vi "downloading_data.vi"(8 "maxDistance":string) -> (0 "Historical indexes":map{string, variant}[](array[numeric]), 1 "Historical standards":map{string, i32}[](array[numeric]), 2 "Current standards [%]":map{string, i32}(c390), 3 "Current indexes":map{string, variant}(c390), 4 "Historical conditions":map{string, i32}[](array[numeric]), 5 "Current conditions":map{string, i32}(c390), 6 "Historical timestamps":map{string, string}[](array[numeric]), 7 "Current timestamps":map{string, string}(c390))   [LabVIEW 2019]
uses:
  <vilib>/Utility/NIReport.llb/Report Type.ctl
  <vilib>/LVH/i3 JSON/JSON Parsing/Get Object Parameter Files/Get Object Parameter - Object.vi
  <vilib>/LVH/i3 JSON/JSON Parsing/Get Object Parameter Files/Get Object Parameter - Array.vi
  <vilib>/LVH/i3 JSON/JSON Parsing/Get Array Value at Index Files/Get Array Value at Index - Object.vi
  <vilib>/Utility/NIReport.llb/NI_report.lvclass
  <vilib>/httpClient/LabVIEWHTTPClient.lvlib
  <vilib>/LVH/i3 JSON/i3-json.lvlib
  <vilib>/Utility/NIReport.llb/NI_ReportGenerationCore.lvlib
  <vilib>/Utility/NIReport.llb/Word/NI_Word.lvclass
panel:
  out "wartości":i32[](array[numeric])
  in  "Window State 2":enum16{"maximized", "minimized", "normal"}(ring)
  in  "Month 2":string[](array[string])=["Jan", "Feb", "Mar", "Apr", "May"]
  in  "Graph Type 2":i32(ring)=51 items=["xlColumnClustered"=51, "xlColumnStacked"=52, "xlColumnStacked100"=53, "xl3DColumnClustered"=54, "xl3DColumnStacked"=55, "xl3DColumnStacked100"=56, "xlBarClustered"=57, "xlBarStacked"=58, "xlBarStacked100"=59, "xl3DBarClustered"=60, "xl3DBarStacked"=61, "xl3DBarStacked100"=62, "xlLineStacked"=63, "xlLineStacked100"=64, "xlLineMarkers"=65, "xlLineMarkersStacked"=66, "xlLineMarkersStacked100"=67, "xlPieOfPie"=68, "xlPieExploded"=69, "xl3DPieExploded"=70, "xlBarOfPie"=71, "xlXYScatterSmooth"=72, "xlXYScatterSmoothNoMarkers"=73, "xlXYScatterLines"=74, "xlXYScatterLinesNoMarkers"=75, "xlAreaStacked"=76, "xlAreaStacked100"=77, "xl3DAreaStacked"=78, "xl3DAreaStacked100"=79, "xlDoughnutExploded"=80, "xlRadarMarkers"=81, "xlRadarFilled"=82, "xlSurface"=83, "xlSurfaceWireframe"=84, "xlSurfaceTopView"=85, "xlSurfaceTopViewWireframe"=86, "xlBubble"=15, "xlBubble3DEffect"=87, "xlStockHLC"=88, "xlStockOHLC"=89, "xlStockVHLC"=90, "xlStockVOHLC"=91, "xlCylinderColClustered"=92, "xlCylinderColStacked"=93, "xlCylinderColStacked100"=94, "xlCylinderBarClustered"=95, "xlCylinderBarStacked"=96, "xlCylinderBarStacked100"=97, "xlCylinderCol"=98, "xlConeColClustered"=99, "xlConeColStacked"=100, "xlConeColStacked100"=101, "xlConeBarClustered"=102, "xlConeBarStacked"=103, "xlConeBarStacked100"=104, "xlConeCol"=105, "xlPyramidColClustered"=106, "xlPyramidColStacked"=107, "xlPyramidColStacked100"=108, "xlPyramidBarClustered"=109, "xlPyramidBarStacked"=110, "xlPyramidBarStacked100"=111, "xlPyramidCol"=112, "xl3DColumn"=-4100, "xlLine"=4, "xl3DLine"=-4101, "xl3DPie"=-4102, "xlPie"=5, "xlXYScatter"=-4169, "xl3DArea"=-4098, "xlArea"=1, "xlDoughnut"=-4120, "xlRadar"=-4151]
  in  "Has Legend? 2":bool
  in  "Relative Humidity 2":dbl[][](array[numeric])=[[0.54, 0.65, 0.56, 0.5, 0.45]]
  in  "Window State":enum16{"maximized", "minimized", "normal"}(ring)
  in  "Month":string[](array[string])=["Jan", "Feb", "Mar", "Apr", "May"]
  in  "Graph Type":i32(ring)=51 items=["xlColumnClustered"=51, "xlColumnStacked"=52, "xlColumnStacked100"=53, "xl3DColumnClustered"=54, "xl3DColumnStacked"=55, "xl3DColumnStacked100"=56, "xlBarClustered"=57, "xlBarStacked"=58, "xlBarStacked100"=59, "xl3DBarClustered"=60, "xl3DBarStacked"=61, "xl3DBarStacked100"=62, "xlLineStacked"=63, "xlLineStacked100"=64, "xlLineMarkers"=65, "xlLineMarkersStacked"=66, "xlLineMarkersStacked100"=67, "xlPieOfPie"=68, "xlPieExploded"=69, "xl3DPieExploded"=70, "xlBarOfPie"=71, "xlXYScatterSmooth"=72, "xlXYScatterSmoothNoMarkers"=73, "xlXYScatterLines"=74, "xlXYScatterLinesNoMarkers"=75, "xlAreaStacked"=76, "xlAreaStacked100"=77, "xl3DAreaStacked"=78, "xl3DAreaStacked100"=79, "xlDoughnutExploded"=80, "xlRadarMarkers"=81, "xlRadarFilled"=82, "xlSurface"=83, "xlSurfaceWireframe"=84, "xlSurfaceTopView"=85, "xlSurfaceTopViewWireframe"=86, "xlBubble"=15, "xlBubble3DEffect"=87, "xlStockHLC"=88, "xlStockOHLC"=89, "xlStockVHLC"=90, "xlStockVOHLC"=91, "xlCylinderColClustered"=92, "xlCylinderColStacked"=93, "xlCylinderColStacked100"=94, "xlCylinderBarClustered"=95, "xlCylinderBarStacked"=96, "xlCylinderBarStacked100"=97, "xlCylinderCol"=98, "xlConeColClustered"=99, "xlConeColStacked"=100, "xlConeColStacked100"=101, "xlConeBarClustered"=102, "xlConeBarStacked"=103, "xlConeBarStacked100"=104, "xlConeCol"=105, "xlPyramidColClustered"=106, "xlPyramidColStacked"=107, "xlPyramidColStacked100"=108, "xlPyramidBarClustered"=109, "xlPyramidBarStacked"=110, "xlPyramidBarStacked100"=111, "xlPyramidCol"=112, "xl3DColumn"=-4100, "xlLine"=4, "xl3DLine"=-4101, "xl3DPie"=-4102, "xlPie"=5, "xlXYScatter"=-4169, "xl3DArea"=-4098, "xlArea"=1, "xlDoughnut"=-4120, "xlRadar"=-4151]
  out "nagłówki":string[](array[string])
  out "longitude":string
  out "latitude":string
  out "Latitude":dbl
  out "Longitude":dbl
  in  "Tab":enum32{"Current", "Historical"}(tab)
  out "body":string
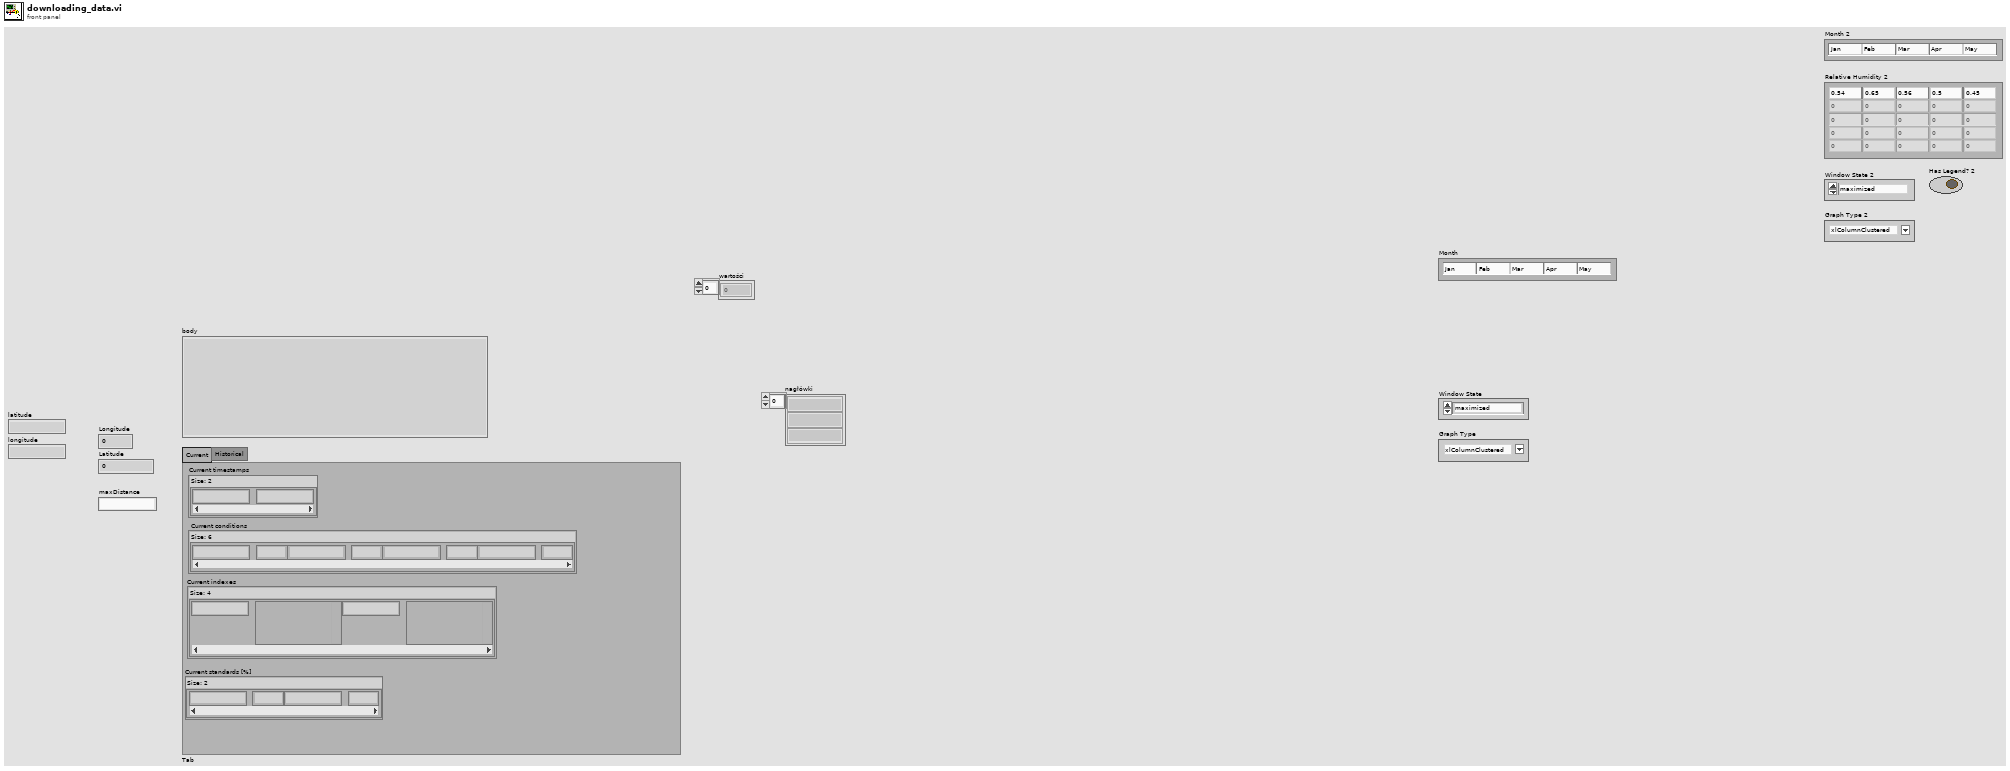
[diagram p1: front panel]
types:
  T1 = cluster{"font style":string, "bold":bool, "italic":bool, "underline":bool, "size":sgl, "color":u32}
  T2 = typedef "NI_ReportGenerationCore.lvlib/Report Type.ctl" = enum16{"HTML", "Word", "Excel"}
  T3 = cluster{"current":cluster{"fromDateTime":string, "tillDateTime":string, "values":cluster{"type and defaults":cluster{"name":string, "value":dbl}, "type and defaults 2":cluster{"name":string, "value":dbl}, "type and defaults 3":cluster{"name":string, "value":dbl}, "type and defaults 4":cluster{"name":string, "value":dbl}, "type and defaults 5":cluster{"name":string, "value":dbl}, "type and defaults 6":cluster{"name":string, "value":dbl}}, "indexes":cluster{"type and defaults":cluster{"name":string, "value":dbl, "level":string, "description":string, "advice":string, "color":string}}, "standards":cluster{"type and defaults":cluster{"name":string, "limit":dbl, "pollutant":string, "percent":dbl}, "type and defaults 2":cluster{"name":string, "limit":dbl, "pollutant":string, "percent":dbl}}}}
  T4 = typedef "LabVIEWHTTPClient.lvlib/ClientHandle.ctl" = refnum<k1>
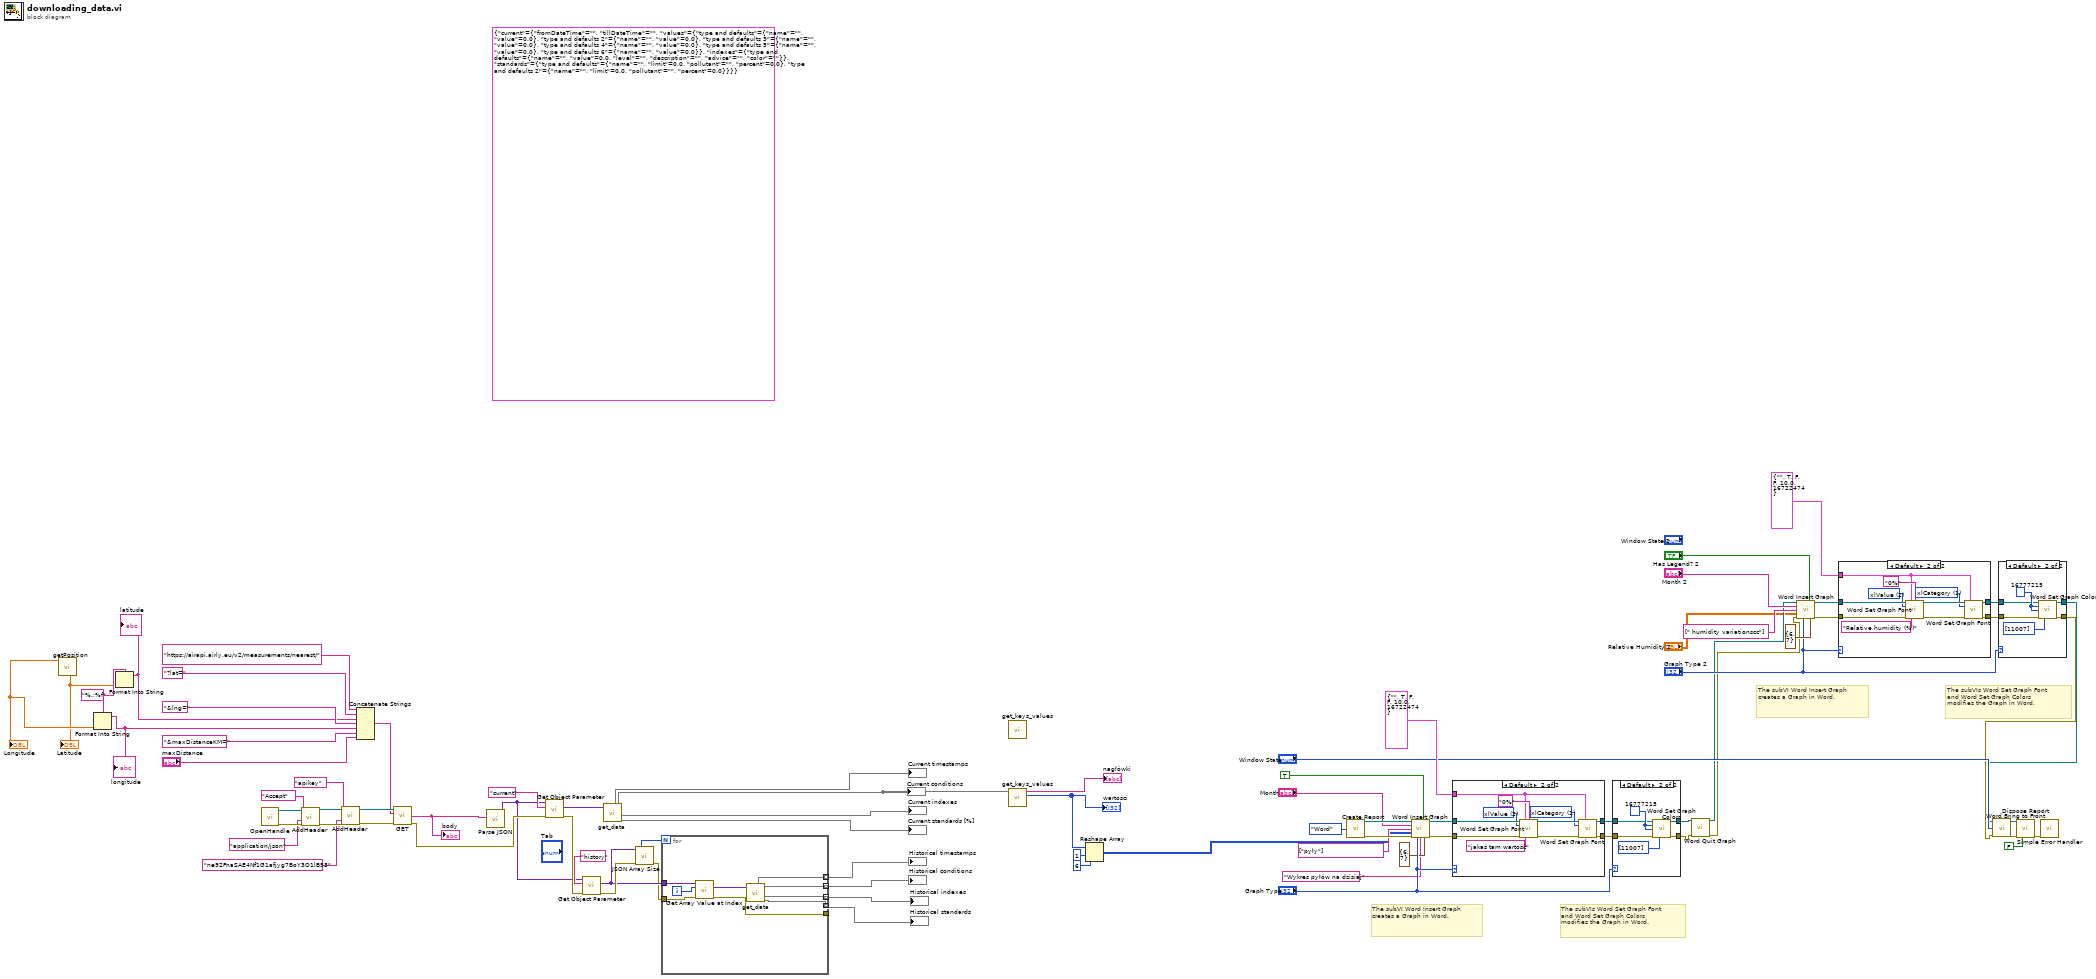
[diagram p0: block diagram]
diagram:
  w45 = "%.;%f" ("format string")
  (unwired) T3 {"current"={"fromDateTime"="", "tillDateTime"="", "values"={"type and defaults"={"name"="", "value"=0.0}, "type and defaults 2"={"name"="", "value"=0.0}, "type and defaults 3"={"name"="", "value"=0.0}, "type and defaults 4"={"name"="", "value"=0.0}, "type and defaults 5"={"name"="", "value"=0.0}, "type and defaults 6"={"name"="", "value"=0.0}}, "indexes"={"type and defaults"={"name"="", "value"=0.0, "level"="", "description"="", "advice"="", "color"=""}}, "standards"={"type and defaults"={"name"="", "limit"=0.0, "pollutant"="", "percent"=0.0}, "type and defaults 2"={"name"="", "limit"=0.0, "pollutant"="", "percent"=0.0}}}} ("type and defaults")
  # "The subVIs Word Set Graph Font \nand Word Set Graph Colors \nmodifies the Graph in Word."
  # "The subVI Word Insert Graph \ncreates a Graph in Word."
  # "The subVIs Word Set Graph Font \nand Word Set Graph Colors \nmodifies the Graph in Word."
  # "The subVI Word Insert Graph \ncreates a Graph in Word."
  n1 = call "getPosition.vi"() -> ("Latitude"=w44:dbl, "Longitude"=w47:dbl)  [unwired: 10 in]
  "Longitude" <- w47
  "Latitude" <- w44
  n2 = Format Into String(format string=w45, w47) -> (resulting string=w48:string)  [unwired: 2 in, 1 out]
  "longitude" <- w48
  n3 = Format Into String(format string=w45, w44) -> (resulting string=w46:string)  [unwired: 2 in, 1 out]
  "latitude" <- w46
  n4 = call <vilib>:"OpenHandle.vi"() -> ("client handle out"=w81:T4, "error out"=w78:errorcluster)  [unwired: 14 in]
  n5 = call <vilib>:"AddHeader.vi"("client handle"=w81, "header"="Accept", "value"="application/json", "error in (no error)"=w78) -> ("client handle out"=w80:T4, "error out"=w77:errorcluster)  [unwired: 10 in]
  n6 = call <vilib>:"AddHeader.vi"("client handle"=w80, "header"="apikey", "value"="ne92FnaSAE4Nf1G1afjyg7BoY3O1lB53", "error in (no error)"=w77) -> ("client handle out"=w79:T4, "error out"=w76:errorcluster)  [unwired: 10 in]
  n7 = Concatenate Strings("https://airapi.airly.eu/v2/measurements/nearest/" ("url"), "?lat=" ("string"), w46, "&lng=" ("string"), w48, "&maxDistanceKM=" ("string"), "maxDistance") -> (w71:string)
  n8 = call <vilib>:"GET.vi"("client handle"=w79, "url"=w71, "error in (no error)"=w76) -> ("body"=w65:string, "error out"=w63:errorcluster)  [unwired: 9 in, 2 out]
  "body" <- w65
  n9 = call <vilib>:"Parse JSON.vi"("JSON String"=w65) -> ("JSON Tree"=w54:variant)  [unwired: 7 in, 3 out]
  n10 = call-poly <vilib>:"Get Object Parameter.vi"("error in (no error)"=w63, "Parameter Name"="current", "JSON Tree In (JSON Object)"=w54) -> ("error out"=w60:errorcluster, "JSON Object"=w61:variant)  [unwired: 5 in, 2 out]
  n11 = call-poly <vilib>:"Get Object Parameter.vi"("error in (no error)"=w60, "Parameter Name"="history", "JSON Tree In (JSON Object)"=w54) -> ("error out"=w58:errorcluster, "JSON Array"=w56:variant)  [unwired: 5 in, 2 out]
  n12 = call "get_data.vi"("JSON"=w61) -> ("Standards [%]"=→"Current standards [%]":map{string, i32}, "Indexes"=→"Current indexes":map{string, variant}, "Conditions"=w7:map{string, i32}, "Timestamps"=→"Current timestamps":map{string, string})  [unwired: 7 in]
  "Current conditions" <- w7
  n13 = call <vilib>:"JSON Array Size.vi"("error in (no error)"=w58, "JSON Tree In (JSON Array)"=w56) -> ("error out"=w55:errorcluster, "Array Size"=w59:i32)  [unwired: 7 in, 1 out]
  n14 = for {
    N: w59 -> [_]
    tunnel: w56 -> [w90]
    tunnel: [w87] -> w53 mode=indexing
    tunnel: [w86] -> w52 mode=indexing
    tunnel: [w85] -> w51 mode=indexing
    tunnel: [w84] -> w57 mode=indexing
    tunnel: w55 -> [w83]
    tunnel: [w82] -> _
    i -> [w89]
    n15 = call-poly <vilib>:"Get Array Value at Index.vi"("error in (no error)"=w83, "Index"=w89, "JSON Tree In (JSON Array)"=w90) -> ("error out"=w82:errorcluster, "JSON Object"=w88:variant)  [unwired: 5 in, 2 out]
    n16 = call "get_data.vi"("JSON"=w88) -> ("Standards [%]"=w85:map{string, i32}, "Indexes"=w86:map{string, variant}, "Conditions"=w87:map{string, i32}, "Timestamps"=w84:map{string, string})  [unwired: 7 in]
  }
  "Historical timestamps" <- w57
  "Historical conditions" <- w53
  "Historical indexes" <- w52
  "Historical standards" <- w51
  n17 = call "get_keys_values.vi"("Conditions"=w7) -> ("wartosci"=w5:i32[], "naglowki"=→"nagłówki":string[])  [unwired: 9 in]
  "wartości" <- w5
  n18 = call "get_keys_values.vi"() -> ()  [unwired: 10 in, 2 out]
  n19 = Reshape Array(w5, 1 ("dimension size"), 6 ("dimension size")) -> (w2:i32[][])
  n20 = call <vilib>:"Create Report.vi"("report type"=Report_Type."Word" ("Report Type")) -> ("report out"=w32:refnum<class "NI_report.lvclass">, "error out"=w33:errorcluster)  [unwired: 13 in]
  n21 = call <vilib>:"Word Insert Graph.vi"("report in"=w32, "has legend? (F)"=TRUE ("Has Legend?"), "column headers"="Month", "row headers"=string[] ["pyły"], "data"=w2, "error in (no error)"=w33, "graph type (col clustered)"="Graph Type", "graph title (\"\")"="Wykres pyłów na dzisiaj" ("graph title (\"\")"), "graph size (5, 5)"=cluster{"height":i32, "width":i32} {"height"=6, "width"=7}) -> ("report out"=w37:refnum<class "NI_report.lvclass">, "error out"=w36:errorcluster)  [unwired: 3 in, 2 out]
  n22 = case shown="Default" "Graph Type" {
    tunnel: w37 -> [w92 w103]
    tunnel: w36 -> [w91 w102]
    tunnel: [w92 w100] -> w34
    tunnel: [w91 w99] -> w35
    tunnel: T1 {"font style"="", "bold"=TRUE, "italic"=FALSE, "underline"=FALSE, "size"=10.0, "color"=16722474} ("axis font") -> [_ w93]
    frame -4151, -4120, -4102, 5, 68..71, 80..82 {
      # "These Graph Types are not supported."
    }
    frame Default {
      w97 = 2 items=["xlCategory"=1, "xlSeriesAxis"=3, "xlValue"=2] ("type")
      w96 = 1 items=["xlCategory"=1, "xlSeriesAxis"=3, "xlValue"=2] ("type")
      n23 = call <vilib>:"Word Set Graph Font.vi"("report in"=w103, "axis font"=w93, "number format (general)"="0%" ("number format (\"\")"), "axis type (category)"=w97, "error in (no error)"=w102, "title (\"\")"="jakaś tam wartość" ("title (\"\")")) -> ("report out"=w101:refnum<class "NI_report.lvclass">, "error out"=w98:errorcluster)  [unwired: 8 in]
      n24 = call <vilib>:"Word Set Graph Font.vi"("report in"=w101, "axis font"=w93, "axis type (category)"=w96, "error in (no error)"=w98) -> ("report out"=w100:refnum<class "NI_report.lvclass">, "error out"=w99:errorcluster)  [unwired: 10 in]
    }
  }
  n25 = case shown="Default" "Graph Type" {
    tunnel: w34 -> [w105 w109]
    tunnel: w35 -> [w104 w108]
    tunnel: [w105 w107] -> w14
    tunnel: [w104 w106] -> w13
    frame 15, 87 {
    }
    frame Default {
      w110 = u32 16777215 ("plot area color")
      n26 = call <vilib>:"Word Set Graph Colors.vi"("report in"=w109, "plot area color (w)"=w110, "graph area color (w)"=w110, "error in (no error)"=w108, "plot colors"=u32[] [11007]) -> ("report out"=w107:refnum<class "NI_report.lvclass">, "error out"=w106:errorcluster)  [unwired: 9 in]
    }
  }
  n27 = call <vilib>:"Word Quit Graph.vi"("report in"=w14, "error in (no error)"=w13) -> ("report out"=w12:refnum<class "NI_report.lvclass">, "error out"=w11:errorcluster)  [unwired: 12 in]
  n28 = call <vilib>:"Word Insert Graph.vi"("report in"=w12, "has legend? (F)"="Has Legend? 2", "column headers"="Month 2", "row headers"=string[] [" humidity variationscc"], "data"="Relative Humidity 2", "error in (no error)"=w11, "graph type (col clustered)"="Graph Type 2", "graph size (5, 5)"=cluster{"height":i32, "width":i32} {"height"=6, "width"=7}) -> ("report out"=w19:refnum<class "NI_report.lvclass">, "error out"=w20:errorcluster)  [unwired: 4 in, 2 out]
  n29 = case shown="Default" "Graph Type 2" {
    tunnel: w19 -> [w113 w124]
    tunnel: w20 -> [w112 w123]
    tunnel: [w113 w121] -> w22
    tunnel: [w112 w120] -> w21
    tunnel: T1 {"font style"="", "bold"=TRUE, "italic"=FALSE, "underline"=FALSE, "size"=10.0, "color"=16722474} ("axis font") -> [_ w114]
    frame -4151, -4120, -4102, 5, 68..71, 80..82 {
      # "These Graph Types are not supported."
    }
    frame Default {
      w118 = 2 items=["xlCategory"=1, "xlSeriesAxis"=3, "xlValue"=2] ("type")
      w117 = 1 items=["xlCategory"=1, "xlSeriesAxis"=3, "xlValue"=2] ("type")
      n30 = call <vilib>:"Word Set Graph Font.vi"("report in"=w124, "axis font"=w114, "number format (general)"="0%" ("number format (\"\")"), "axis type (category)"=w118, "error in (no error)"=w123, "title (\"\")"="Relative humidity (%)" ("title (\"\")")) -> ("report out"=w122:refnum<class "NI_report.lvclass">, "error out"=w119:errorcluster)  [unwired: 8 in]
      n31 = call <vilib>:"Word Set Graph Font.vi"("report in"=w122, "axis font"=w114, "axis type (category)"=w117, "error in (no error)"=w119) -> ("report out"=w121:refnum<class "NI_report.lvclass">, "error out"=w120:errorcluster)  [unwired: 10 in]
    }
  }
  n32 = case shown="Default" "Graph Type 2" {
    tunnel: w22 -> [w126 w130]
    tunnel: w21 -> [w125 w129]
    tunnel: [w126 w128] -> w9
    tunnel: [w125 w127] -> w8
    frame 15, 87 {
    }
    frame Default {
      w131 = u32 16777215 ("plot area color")
      n33 = call <vilib>:"Word Set Graph Colors.vi"("report in"=w130, "plot area color (w)"=w131, "graph area color (w)"=w131, "error in (no error)"=w129, "plot colors"=u32[] [11007]) -> ("report out"=w128:refnum<class "NI_report.lvclass">, "error out"=w127:errorcluster)  [unwired: 9 in]
    }
  }
  n34 = call <vilib>:"Word Bring to Front.vi"("report in"=w9, "window state (maximized)"="Window State", "error in (no error)"=w8) -> ("report out"=w31:refnum<class "NI_report.lvclass">, "error out"=w29:errorcluster)  [unwired: 11 in]
  n35 = call-dynamic "Dispose Report.vi"("report in"=w31, "error in (no error)"=w29, "close report? (T)"=FALSE ("Close Report? (T)")) -> ("error out"=w25:errorcluster)  [unwired: 12 in]
  n36 = call <vilib>:"Simple Error Handler.vi"("error in (no error)"=w25) -> ()  [unwired: 4 in, 5 out]
